vi "Read Process.vi"(11 "Process State in":refnum<class "Process State.lvclass">) -> (2 "Process Enqueuer":refnum<class "Message Enqueuer.lvclass">, 3 "Process State out":refnum<class "Process State.lvclass">)   [LabVIEW 2012, in "Process States.lvlib" / "Process State.lvclass"]
doc: "Returns the enqueuer for the nested Process Actor."
uses:
  Process State.lvclass
  <vilib>/ActorFramework/Message Enqueuer/Message Enqueuer.lvclass
  Process State.lvclass/Process State.ctl
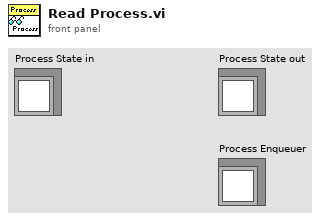
[diagram p1: front panel]
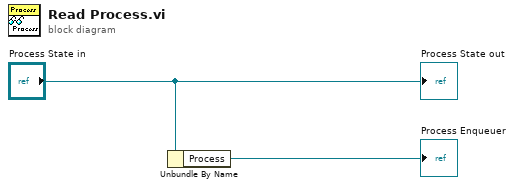
[diagram p0: block diagram]
diagram:
  n1 = Unbundle By Name("Process State in") -> ("Process"=→"Process Enqueuer":refnum<class "Message Enqueuer.lvclass">)
  "Process State out" <- "Process State in"
